vi "RefreshSystemConfigurationUI.vi"(8 "error in (no error)":errorcluster, 11 "TestSetup in":refnum<class "TestSetup.lvclass">) -> (0 "error out":errorcluster, 3 "TestSetup out":refnum<class "TestSetup.lvclass">)   [LabVIEW 2019, in "TestSetup.lvlib" / "TestSetup.lvclass"]
uses:
  TestSetup.lvclass
  C:/Program Files (x86)/National Instruments/LabVIEW 2019/vi.lib/NI/Event Source Actor/Event Source/Event Source/Event Source.lvclass
  TestSetup.lvclass/TestSetup.ctl
  TestConfiguration.lvclass
  C:/Program Files (x86)/National Instruments/LabVIEW 2019/vi.lib/NI/Event Source Actor/Event Source/Event/Event.lvclass
  <vilib>/NI/Event Source Actor/Event Source/Event/Event.lvclass/Event.ctl
  <vilib>/Utility/file.llb/Read Delimited Spreadsheet (string).vi
  SystemSetup/SystemSetup/SystemSetup.lvclass
  <vilib>/NI/Event Source Actor/Event Source/Event/Event.lvclass
  <vilib>/NI/Event Source Actor/Event Source/Event Source/Event Source.lvclass
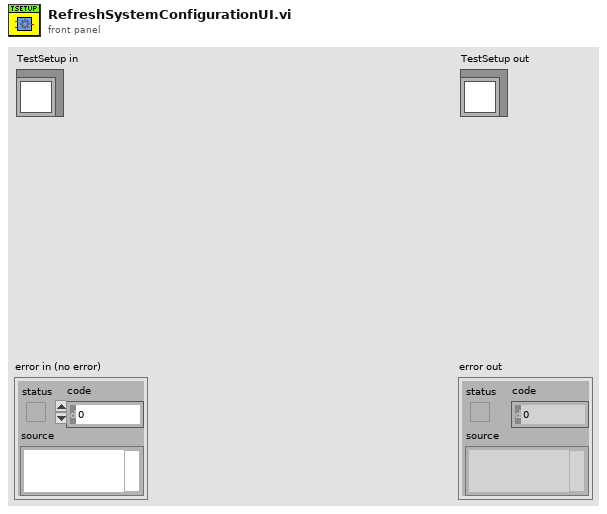
[diagram p1: front panel]
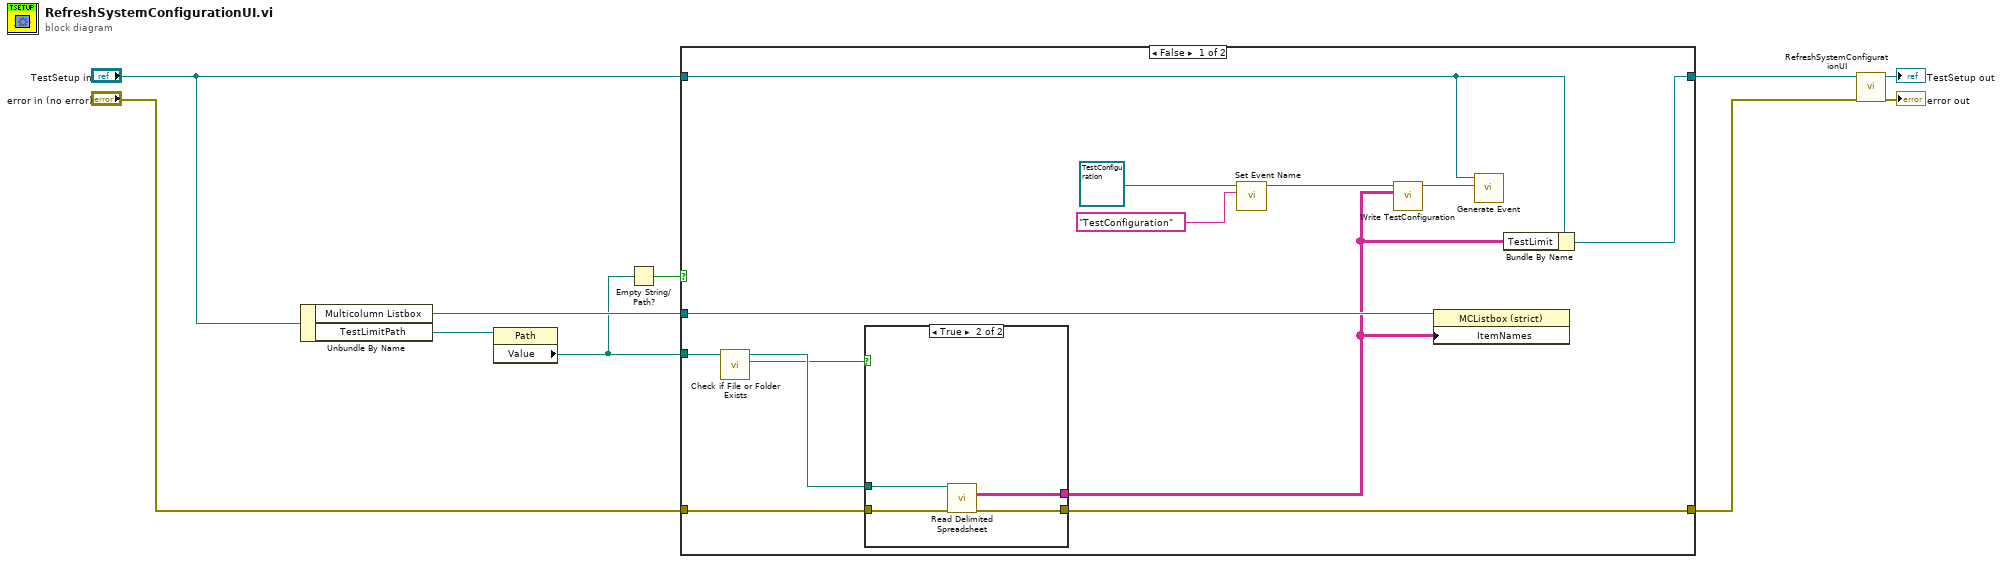
[diagram p0: block diagram]
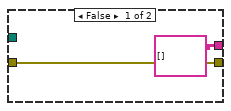
[diagram p2: hidden frame]
diagram:
  n1 = Unbundle By Name("TestSetup in") -> ("Multicolumn Listbox"=w8:refnum<vi>, "TestLimitPath"=w7:refnum<vi>)
  n2 = property class="Path"(reference=w7) -> ("Value"=w6:path)  [unwired: 1 in, 2 out]
  n3 = Empty String/Path?(string/path=w6) -> (empty?=w5:bool)
  n4 = case shown="False" w5 {
    tunnel: "error in (no error)" -> [w15 w30]
    tunnel: [w13 w30] -> w1
    tunnel: w8 -> [w23 _]
    tunnel: "TestSetup in" -> [w18 w31]
    tunnel: [w17 w31] -> w2
    tunnel: w6 -> [w16 _]
    frame False {
      n5 = call <vilib>:"Check if File or Folder Exists.vi"("path"=w16) -> ("file or folder exists?"=w11:bool, "dup path"=w12:path)  [unwired: 8 in, 1 out]
      n6 = case shown="True" w11 {
        tunnel: w15 -> [w25 w29]
        tunnel: [string[][] [] ("all rows") w28] -> w14
        tunnel: [w25 w27] -> w13
        tunnel: w12 -> [_ w26]
        frame False {
        }
        frame True {
          n7 = call-poly <vilib>:"Read Delimited Spreadsheet.vi"("file path (dialog if empty)"=w26, "error in (no error)"=w29) -> ("all rows"=w28:string[][], "error out"=w27:errorcluster)  [unwired: 8 in, 4 out]
        }
      }
      n8 = call <vilib>:"Set Event Name.vi"("Name (Generic)"="TestConfiguration", "Event In"=refnum<class "TestConfiguration.lvclass"> refnum ("TestSetup.lvlib:TestConfiguration.lvclass")) -> ("Event Out"=w20:refnum<class "TestConfiguration.lvclass">)  [unwired: 9 in]
      n9 = call-dynamic "Write TestConfiguration.vi"("TestLimit"=w14, "TestConfiguration in"=w20) -> ("TestConfiguration out"=w19:refnum<class "TestConfiguration.lvclass">)  [unwired: 8 in, 1 out]
      n10 = property class="MCListbox (strict)"(reference=w23, "ItemNames"=w14) -> ()  [unwired: 1 in, 2 out]
      n11 = call <vilib>:"Generate Event.vi"("Event"=w19, "Event Source In"=w18) -> ()  [unwired: 8 in, 2 out]
      n12 = Bundle By Name(cluster=w18, "TestLimit"=w14) -> (w17:refnum<class "TestSetup.lvclass">)
    }
    frame True {
    }
  }
  n13 = call-parent "RefreshSystemConfigurationUI.vi"("error in (no error)"=w1, "SystemSetup in"=w2) -> ("error out"=→"error out":errorcluster, "SystemSetup out"=→"TestSetup out":refnum<class "TestSetup.lvclass">)  [unwired: 8 in]
